vi "N-Parametric Double FFT Mesurament (MAX BIN DETECT) SLOW Test.vi"() -> ()   [LabVIEW 2014]
uses:
  <vilib>/Platform/TimedLoop/XDataNode/timing_clust.ctl
  <vilib>/Platform/TimedLoop/XDataNode/nitl_modes.ctl
  <vilib>/Platform/TimedLoop/XDataNode/wakeup.ctl
  <vilib>/rvi/Analysis/measure/FFT/simModelSupport/niFPGA FFT Streaming Sim Properties.ctl
  <vilib>/rvi/Analysis/measure/FFT/simModelSupport/niFPGA FFT Sim Stream Group Properties.ctl
  <vilib>/rvi/Analysis/measure/FFT/simModelSupport/niFPGA FFT Sim Types.ctl
  <vilib>/rvi/Analysis/measure/FFT/simModelSupport/niFpgaFFTSimArithmeticProperties.ctl
  <vilib>/rvi/Analysis/measure/FFT/simModelSupport/niFpgaFFTSimDfxp.ctl
  <vilib>/fxp/LVFixedPointQuantizationPolicyTypeDef.ctl
  <vilib>/rvi/Analysis/measure/FFT/XNode/niFpgaFFTButterflyDelays.ctl
  <vilib>/rvi/Emulation/niFpgaSctlEmulationGetInTimedLoop.vi
  <vilib>/rvi/Emulation/niFpgaEmulationReportErrorSimple.vi
  <vilib>/rvi/Emulation/niFpgaGetClockAttributes.vi
  <vilib>/rvi/Emulation/niFpgaCriticalErrorInLSC.vi
  <vilib>/rvi/Emulation/niFpgaEmulationIsFPGAContextNoSignature.vi
  <vilib>/rvi/errors/niFpgaSetErrorForExecOnDevCompSimple.vi
  <vilib>/rvi/eio/common/nirviEmuReportErrorAndStop.vi
  <vilib>/rvi/DataTransferAndStorage/Container/Common/niFpgaContainerGetUniqueNameForEmu.vi
  <vilib>/rvi/FIFO/Fifo_Resource/nirvififoEmulationSetSize.vi
  <vilib>/rvi/FIFO/Fifo_Resource/nirviFifoEmulationQueueMgr.vi
  <instcachedir>/0/nirviFifoEmulationQueueMgr_E5CAEC123FF24DC58D834DCA3CDAA9B5.lvgen/nirviFifoEmulationQueueMgr_E5CAEC123FF24DC58D834DCA3CDAA9B5_014.vi
  <vilib>/rvi/FIFO/Fifo_Resource/nirvififoEmulationCreateLock.vi
  <vilib>/rvi/Emulation/niFpgaProcessEmulError.vi
  <vilib>/rvi/FIFO/Fifo_Resource/nirvififoEmulationObtainLock.vi
  <vilib>/rvi/FIFO/Fifo_Resource/nirvififoEmulationReleaseLock.vi
  <vilib>/rvi/occurrence/nirviWaitOnOccurrenceBase.vi
  <vilib>/rvi/errors/nirviReportUnexpectedCaseInternalError.vi
  <vilib>/rvi/errors/nirviReportUnexpectedCaseInternalError (U32).vi
  <vilib>/rvi/Memory/Memory_Emulation/niFpgaMemoryEmulationCacheClearOnFirstRun.vi
  <vilib>/rvi/Memory/Memory_Emulation/nirvimemoryEmulationManagerCache_MakeExclusive.vi
  <vilib>/rvi/Memory/Memory_Emulation/niFpgaMemoryEmulationValidateCache.vi
  <vilib>/rvi/Memory/Memory_Emulation/nirvimemoryEmulationManagerCache_InsertValue.vi
  <vilib>/Utility/error.llb/Clear Errors.vi
  <vilib>/rvi/Memory/Memory_Emulation/nirvimemoryEmulationManagerCache_ReleaseExclusive.vi
  <vilib>/rvi/Memory/Memory_Emulation/nirvimemoryEmulationManagerCache_GetValue.vi
  <vilib>/rvi/Memory/Memory_Emulation/nirvimemoryEmulationManagerCache_SetValue.vi
  <instcachedir>/0/nirviFifoEmulationQueueMgr_E5CAEC123FF24DC58D834DCA3CDAA9B5.lvgen/nirviFifoEmulationQueueMgr_E5CAEC123FF24DC58D834DCA3CDAA9B5_010.vi
  <vilib>/rvi/FIFO/Fifo_Resource/nirvififoEmulationDetermineInputValidOut.vi
  <vilib>/rvi/Memory/Memory_Emulation/nirvimemoryFastEmulation.vi
  <vilib>/rvi/Memory/Memory_Emulation/nirvimemoryEmulation.vi
  <vilib>/rvi/Analysis/measure/FFT/simModelSupport/niFpgaFFTSimModelStreamingCore.vi
  <vilib>/rvi/eio/common/nirviEmuTemplateMethod_errors.vi
  <vilib>/Platform/TimedLoop/XDataNode/XDataNode.xnode
  <vilib>/rvi/DataTransferAndStorage/Container/XNode/niFpgaContainer.xnode
  <vilib>/rvi/FIFO/Fifo_Resource/nirvififoEmulationRead.vi
  <vilib>/rvi/DataTransferAndStorage/Register/Emulation/niFpgaRegisterEmulation.vi
  <vilib>/rvi/FIFO/Fifo_Resource/nirvififoEmulationWrite.vi
  <vilib>/rvi/FIFO/Fifo_Resource/nirvififoEmulationGetNumberOfElementsToWrite.vi
  <vilib>/rvi/Analysis/measure/FFT/XNode/niFpgaFFT.xnode
  <vilib>/eio/EIOMethodNode/EIOMethodNode.xnode
  <vilib>/Platform/TimedLoop/XDataNode/XDNodeRunTimeDep.lvlib
panel:
  in  "First bin":i32=5
  in  "Last bin":i32=255
  in  "Hanning window":bool=TRUE
  in  "n":u32=5
  in  "Latency points":u32
  in  "lower limit 2":u32=682
  in  "lower limit 1":u32=57
  in  "upper limit 2":u32=1193
  in  "upper limit 1":u32=568
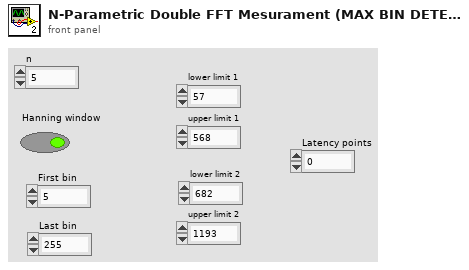
[diagram p1: front panel]
types:
  T1 = typedef "XDNodeRunTimeDep.lvlib/timing_clust.ctl" = cluster{"Expected End [f-1]":u64, "Actual End [f-1]":u64, "Finished Late? [f-1]":bool, "Expected End [i-1]":u64, "Actual End [i-1]":u64, "Finished Late? [i-1]":bool, "Expected Start [i]":u64, "Actual Start [i]":u64, "Expected Start [f]":u64, "Actual Start [f]":u64, "Source Name":string, "Structure Name":string, "Period":i64, "Deadline":i64, "Offset":i64, "Start":i64, "Priority":i32, "Timeout":i32, "Mode":T2, "Wakeup Reason":T3, "Error":errorcluster, "Source Type":string, "Secondary Source Type":string, "Global End Time":u64, "Global Start Time":u64, "Frame Duration":u64, "Iteration Duration":u64, "Assigned CPU":i32, "I/O Scan Engine Mode":u32}
  T2 = typedef "XDNodeRunTimeDep.lvlib/nitl_modes.ctl" = enum32{"No Change", "Process missed periods, maintain original phase", "Discard missed periods, maintain original phase", "Process missed periods, ignore original phase", "Discard missed periods, ignore original phase"}
  T3 = typedef "XDNodeRunTimeDep.lvlib/wakeup.ctl" = enum32{"Normal", "Aborted", "Asynchronous wakeup", "Timing source error", "Timed loop error", "Timeout"}
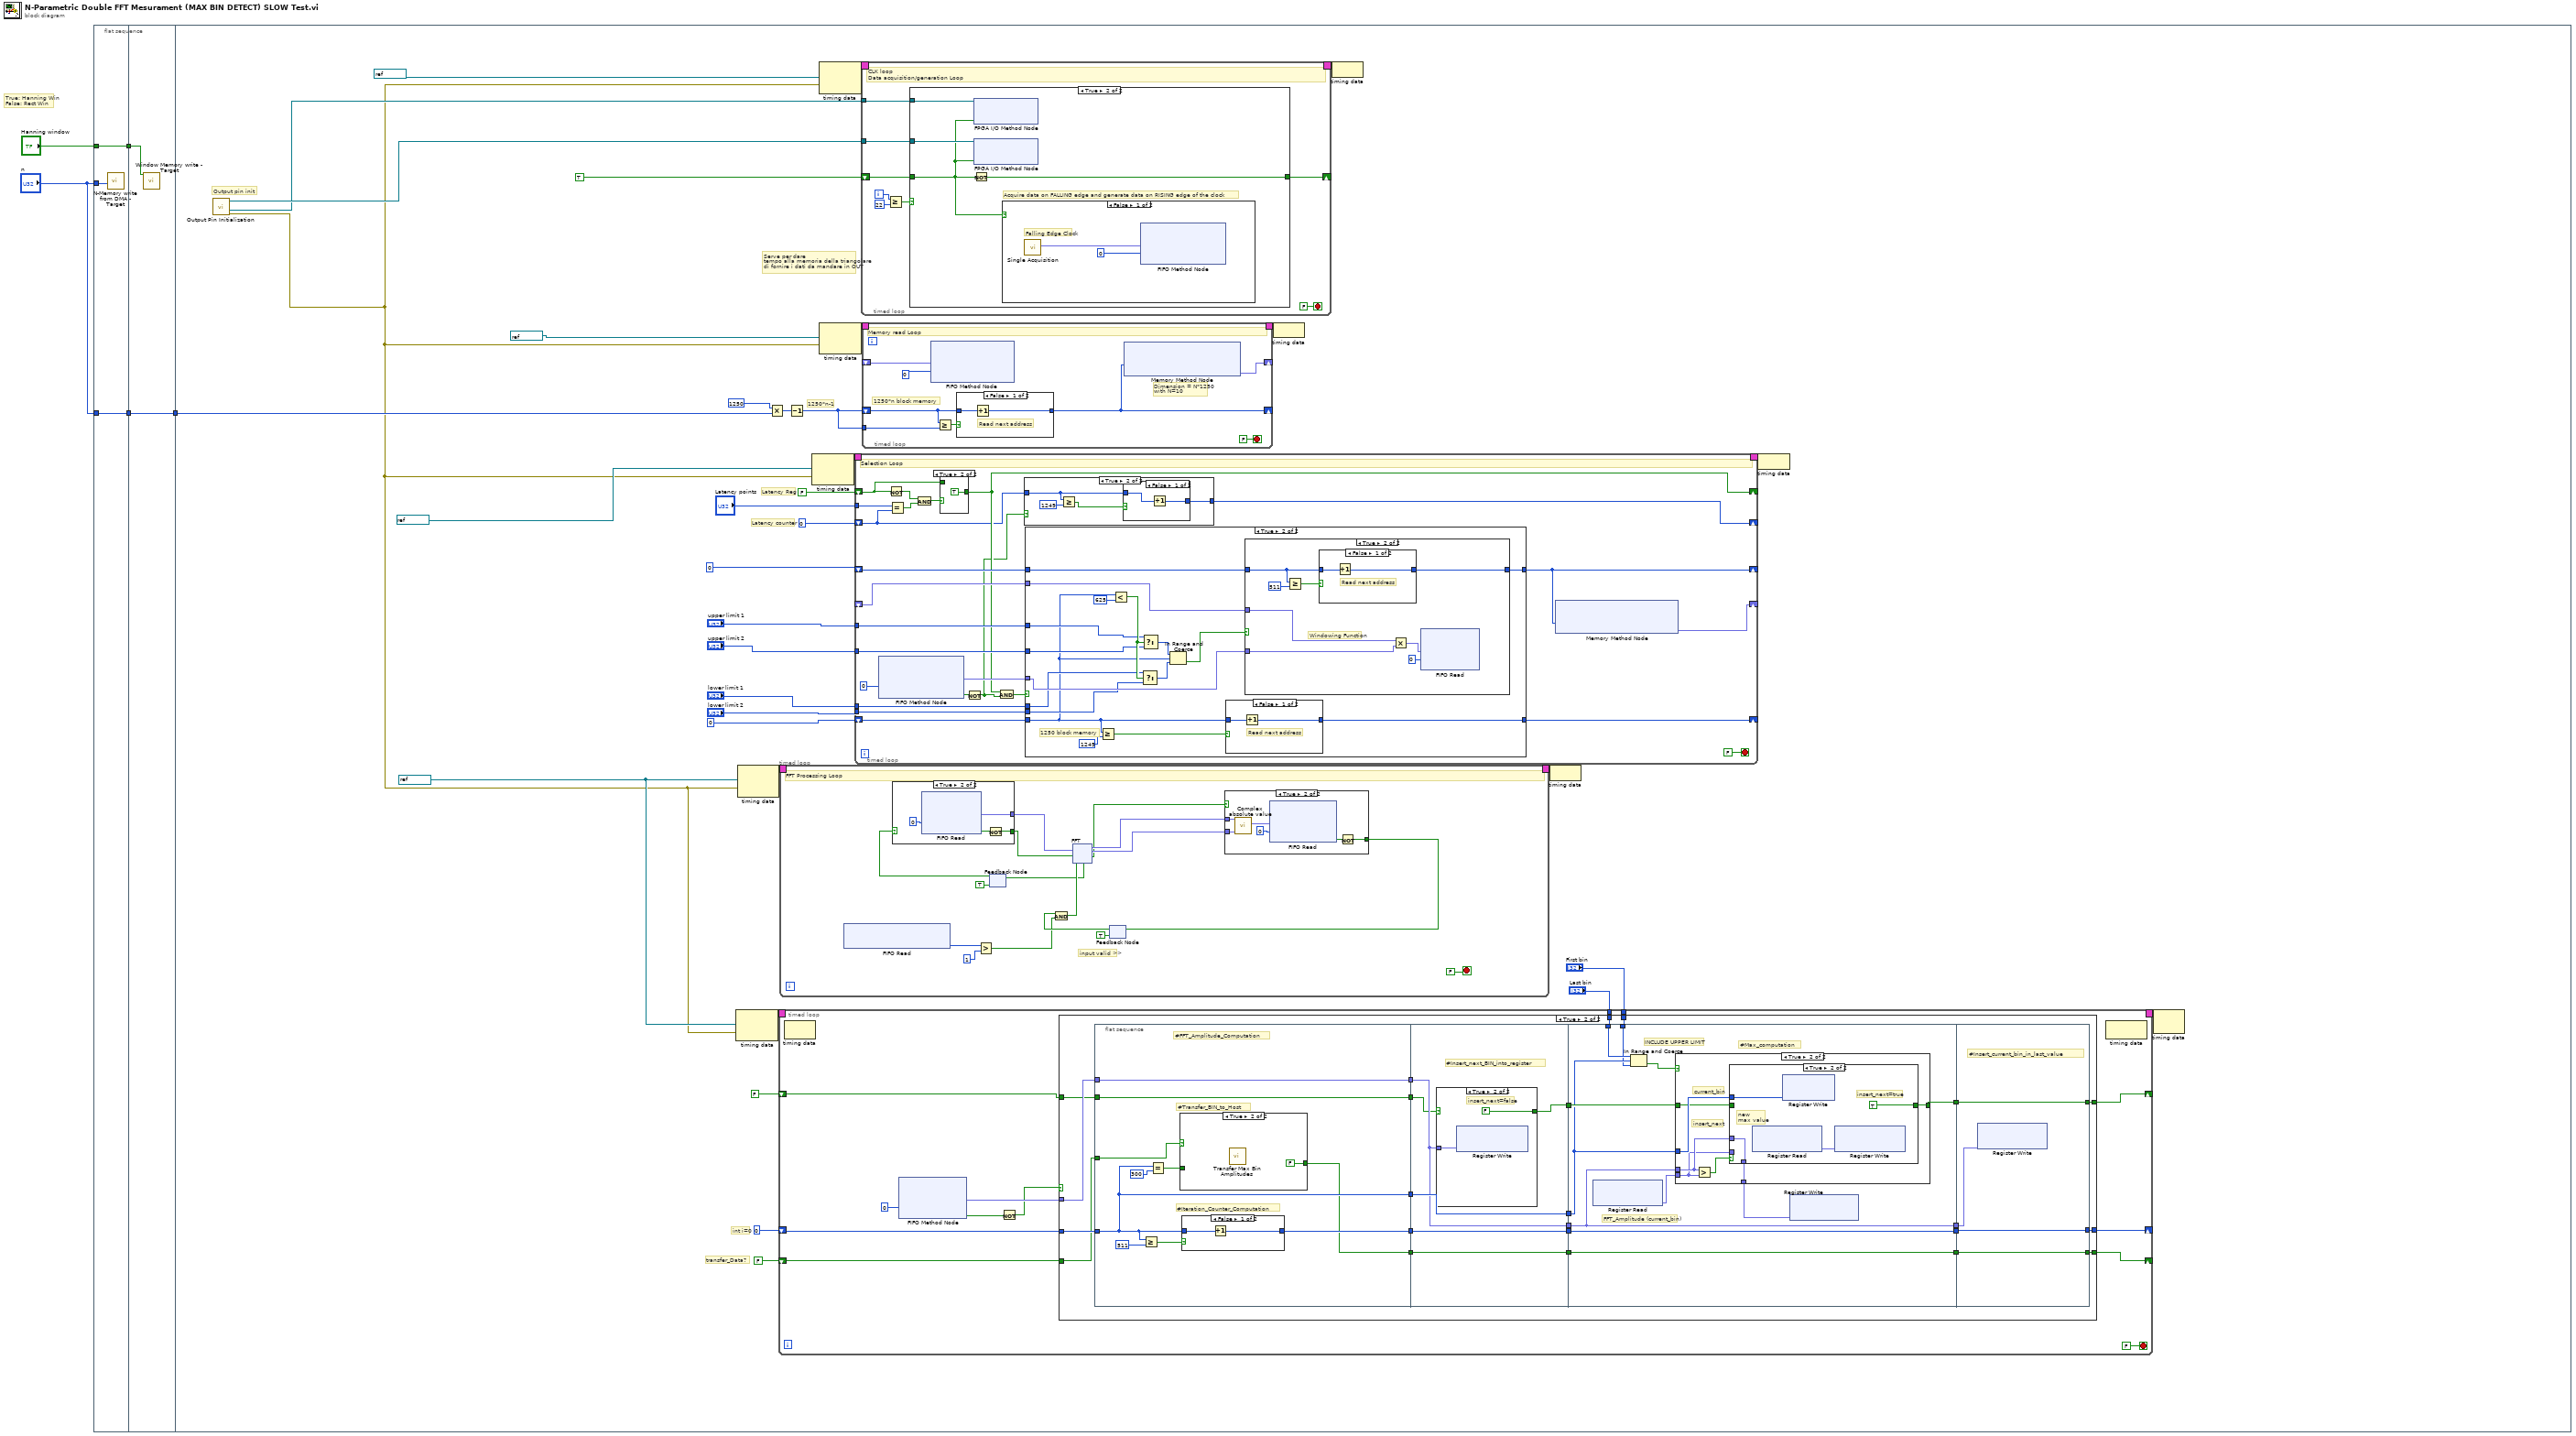
[diagram p0: block diagram]
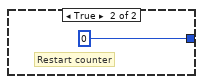
[diagram p4: hidden frame]
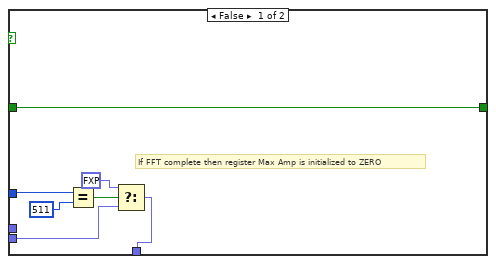
[diagram p6: hidden frame]
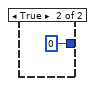
[diagram p9: hidden frame]
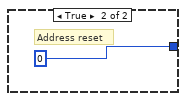
[diagram p13: hidden frame]
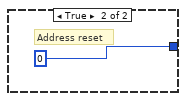
[diagram p14: hidden frame]
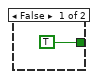
[diagram p15: hidden frame]
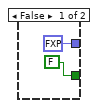
[diagram p16: hidden frame]
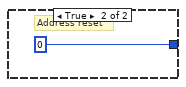
[diagram p17: hidden frame]
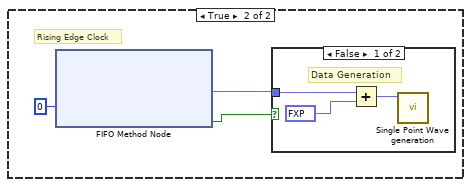
[diagram p19: hidden frame]
diagram:
  # "True: Hanning Win\nFalse: Rect Win"
  n1 = flat-sequence {
    tunnel: "n" -> [w8]
    tunnel: "n" -> [w7]
    tunnel: [w7] -> w4
    tunnel: "Hanning window" -> [w6]
    tunnel: [w6] -> w1
    tunnel: w4 -> [w10]
    tunnel: [w10] -> w3
    tunnel: w1 -> [w9]
    tunnel: w3 -> [w20]
    frame #0 {
      n2 = call "N-Memory write from DMA - Target.vi"("n"=w8) -> ()  [unwired: 11 in]
    }
    frame #1 {
      n3 = call "Window Memory write - Target.vi"("Hanning window"=w9) -> ()  [unwired: 11 in]
    }
    frame #2 {
      w12 = refnum<k21> "30MHz" ("Source Name")
      # "transfer_Data?"
      # "int i=0"
      # "1250*n-1"
      # "Serve per dare\ntempo alla memoria della triangolare\ndi fornire i dati da mandare in OUT"
      # "Latency counter"
      # "Latency Reg"
      # "Output pin init"
      n4 = call "Output Pin Initialization.vi"() -> ("error out"=w11:errorcluster, "I/O Out Clock DAC (pin16)"=w34:refnum<k21>, "I/O Out Clock ADC (pin17)"=w35:refnum<k21>)  [unwired: 8 in]
      n5 = node-c288(w12, w11) -> (w19:T1)
      n6 = node-c288(w12, w11) -> (w42:T1)
      n7 = Multiply(x=u32 1250, y=w20) -> (x*y=w22:u32)
      n8 = timed-loop {
        shift-right: [w56] -> _
        shift-left: FALSE -> [w55]
        shift-right: [w54] -> _
        shift-left: 0 ("Timeout") -> [w57]
        shift-right: [w53] -> _
        shift-left: FALSE -> [w49]
        tunnel: "Last bin" -> [w51]
        tunnel: "First bin" -> [w50]
        timing: w19 -> [_]
        timing-out: [_] -> w18
        stop <- FALSE stop-if-true
        n9 = node-c288() -> ()  [unwired: 1 in, 1 out]
        n10 = xnode ("FIFO Method Node")("Timeout"=0) -> ("Element"=w58:fxp<+,44,44>, "Timed Out?"=w59:bool)  [unwired: 1 in, 1 out]
        n11 = Not(x=w59) -> (.not. x?=w52:bool)
        n12 = case shown="True" w52 {
          tunnel: w58 -> [_ w87]
          tunnel: w57 -> [w64 w85]
          tunnel: [w64 w72] -> w54
          tunnel: w55 -> [w63 w79]
          tunnel: [w63 w74] -> w56
          tunnel: w51 -> [_ w71]
          tunnel: w50 -> [_ w70]
          tunnel: w49 -> [w62 w69]
          tunnel: [w62 w68] -> w53
          frame False {
            # "Data are NOT ready in FIFO"
          }
          frame True {
            n13 = flat-sequence {
              tunnel: w87 -> [w88]
              tunnel: [w88] -> w86
              tunnel: w85 -> [w92]
              tunnel: [w97] -> w84
              tunnel: [w92] -> w81
              tunnel: [w94] -> w80
              tunnel: w79 -> [w94]
              tunnel: w69 -> [w91]
              tunnel: [w89] -> w67
              tunnel: w86 -> [w106]
              tunnel: w84 -> [w108]
              tunnel: [w108] -> w83
              tunnel: w81 -> [w107]
              tunnel: w80 -> [w104]
              tunnel: [w107] -> w78
              tunnel: [w106] -> w77
              tunnel: [w103] -> w76
              tunnel: w67 -> [w105]
              tunnel: [w105] -> w66
              tunnel: w83 -> [w122]
              tunnel: [w122] -> w82
              tunnel: w78 -> [w117]
              tunnel: w77 -> [w119]
              tunnel: w76 -> [w120]
              tunnel: [w119] -> w75
              tunnel: [w118] -> w73
              tunnel: w71 -> [w114]
              tunnel: w70 -> [w113]
              tunnel: w66 -> [w112]
              tunnel: [w112] -> w65
              tunnel: w82 -> [w144]
              tunnel: w75 -> [w146]
              tunnel: w73 -> [w145]
              tunnel: [w145] -> w74
              tunnel: [w144] -> w72
              tunnel: [w143] -> w68
              tunnel: w65 -> [w143]
              frame #0 {
                # "#Transfer_BIN_to_Host"
                # "#Iteration_Counter_Computation"
                # "#FFT_Amplitude_Computation"
                n14 = Greater Or Equal?(x=w92, y=511) -> (x >= y?=w95:bool)
                n15 = Equal?(x=w92, y=300) -> (x = y?=w90:bool)
                n16 = case shown="True" w91 {
                  tunnel: w90 -> [w98 _]
                  tunnel: [w98 FALSE] -> w89
                  frame False {
                    # "FFT Comp is NOT finished"
                  }
                  frame True {
                    n17 = call "Transfer Max Bin Amplitudes.vi"() -> ()  [unwired: 12 in]
                  }
                }
                n18 = case shown="False" w95 {
                  tunnel: w92 -> [w100 _]
                  tunnel: [w101 0 ("Timeout")] -> w97
                  frame False {
                    n19 = Increment(x=w100) -> (x+1=w101:i32)
                  }
                  frame True {
                    # "Restart counter"
                  }
                }
              }
              frame #1 {
                # "#Insert_next_BIN_into_register"
                n20 = case shown="True" w104 {
                  selector: w104 -> [w109 _]
                  tunnel: [w109 FALSE] -> w103
                  tunnel: w106 -> [_ w110]
                  frame False {
                  }
                  frame True {
                    # "insert_next=false"
                    n21 = xnode ("Register Write")("Data"=w110) -> ()  [unwired: 1 in, 1 out]
                  }
                }
              }
              frame #2 {
                # "INCLUDE UPPER LIMIT"
                # "FFT_Amplitude (current_bin)"
                # "#Max_computation"
                n22 = xnode ("Register Read")() -> ("Data"=w116:fxp<+,44,44>)  [unwired: 1 in, 1 out]
                n23 = In Range and Coerce(upper limit=w114, x=w117, lower limit=w113) -> (In Range?=w121:bool)  [unwired: 1 out]
                n24 = case shown="True" w121 {
                  tunnel: w119 -> [_ w135]
                  tunnel: w117 -> [w127 w134]
                  tunnel: w120 -> [w129 w133]
                  tunnel: [w129 w132] -> w118
                  tunnel: w116 -> [w125 w130]
                  tunnel: [w123 w131] -> w115
                  frame False {
                    # "If FFT complete then register Max Amp is initialized to ZERO"
                    n25 = Equal?(x=w127, y=511) -> (x = y?=w128:bool)
                    n26 = Select(t=fxp<+,44,44> 0.0, s=w128, f=w125) -> (s? t:f=w123:fxp<+,44,44>)
                  }
                  frame True {
                    # "insert_next"
                    # "current_bin"
                    n27 = Greater?(x=w135, y=w130) -> (0:w136:bool)
                    n28 = case shown="True" w136 {
                      tunnel: w135 -> [_ w140]
                      tunnel: w134 -> [_ w142]
                      tunnel: w133 -> [w138 _]
                      tunnel: [w138 TRUE] -> w132
                      tunnel: [w137 w140] -> w131
                      tunnel: w130 -> [w137 _]
                      frame False {
                        # "Old value is re-written"
                      }
                      frame True {
                        # "new\nmax value"
                        # "insert_next=true"
                        n29 = xnode ("Register Read")() -> ("Data"=w139:fxp<+,44,44>)  [unwired: 1 in, 1 out]
                        n30 = xnode ("Register Write")("Data"=w142) -> ()  [unwired: 1 in, 1 out]
                        n31 = xnode ("Register Write")("Data"=w139) -> ()  [unwired: 1 in, 1 out]
                      }
                    }
                  }
                }
                n32 = xnode ("Register Write")("Data"=w115) -> ()  [unwired: 1 in, 1 out]
              }
              frame #3 {
                # "#Insert_current_bin_in_last_value"
                n33 = xnode ("Register Write")("Data"=w146) -> ()  [unwired: 1 in, 1 out]
              }
            }
          }
        }
        n34 = node-c288() -> ()  [unwired: 1 in, 1 out]
      }
      n35 = timed-loop {
        timing: w42 -> [_]
        timing-out: [_] -> w41
        stop <- FALSE stop-if-true
        # "input valid >>"
        # "FFT Processing Loop"
        n36 = xnode ("FIFO Read")() -> ("Number of Elements to Write"=w227:u32)  [unwired: 1 in, 1 out]
        n37 = Greater?(x=w227, y=u32 1) -> (0:w228:bool)
        n38 = feedback #1(TRUE ("ready for input")) -> (w242:bool)
        n39 = case shown="True" w242 {
          tunnel: [FALSE w281] -> w232
          tunnel: [fxp<+/-,12,12> 0.0 ("Element") w278] -> w233
          frame False {
          }
          frame True {
            n40 = xnode ("FIFO Read")("Timeout"=0) -> ("Element"=w278:fxp<+/-,12,12>, "Timed Out?"=w280:bool)  [unwired: 1 in, 1 out]
            n41 = Not(x=w280) -> (.not. x?=w281:bool)
          }
        }
        n42 = feedback #2(TRUE) -> (w238:bool)
        n43 = Compound Arithmetic op=AND(w238, w228) -> (w237:bool)
        n44 = xnode "FFT"("real data in"=w233, "input valid"=w232, "ready for output"=w237) -> ("ready for input"=w236:bool, "real data out"=w235:fxp<+/-,22,22>, "imaginary data out"=w234:fxp<+/-,22,22>, "output valid"=w231:bool)  [unwired: 2 in, 1 out]
        n45 = feedback-in #1(w236) -> ()
        n46 = case shown="True" w231 {
          tunnel: w235 -> [_ w275]
          tunnel: w234 -> [_ w274]
          tunnel: [TRUE w273] -> w230
          frame False {
          }
          frame True {
            n47 = call "Complex absolute value.vi"("Im"=w274, "Re"=w275) -> ("Square Absolute Value"=w272:fxp<+,44,44>)  [unwired: 9 in]
            n48 = xnode ("FIFO Read")("Element"=w272, "Timeout"=0) -> ("Timed Out?"=w270:bool)  [unwired: 1 in, 1 out]
            n49 = Not(x=w270) -> (.not. x?=w273:bool)
          }
        }
        n50 = feedback-in #2(w230) -> ()
      }
      n51 = Decrement(x=w22) -> (x-1=w21:u32)
      n52 = node-c288(refnum<k21> "30MHz" ("Source Name"), w11) -> (w40:T1)
      n53 = node-c288(refnum<k21> "60MHz" ("Source Name"), w11) -> (w46:T1)
      n54 = node-c288(refnum<k21> "30MHz" ("Source Name"), w11) -> (w44:T1)
      n55 = timed-loop {
        timing: w40 -> [_]
        timing-out: [_] -> w39
        shift-right: [w174] -> _
        shift-left: u32 0 -> [w161]
        tunnel: "upper limit 1" -> [w170]
        tunnel: "upper limit 2" -> [w169]
        tunnel: "lower limit 1" -> [w168]
        tunnel: "lower limit 2" -> [w167]
        shift-right: [w163] -> _
        shift-left: u32 0 -> [w166]
        shift-right: [w164] -> _
        shift-left: _ -> [w165]
        shift-right: [w155] -> _
        shift-left: FALSE -> [w156]
        tunnel: "Latency points" -> [w160]
        shift-right: [w153] -> _
        shift-left: u32 0 -> [w152]
        stop <- FALSE stop-if-true
        # "Selection Loop"
        n56 = xnode ("FIFO Method Node")("Timeout"=0) -> ("Element"=w172:fxp<+/-,12,12>, "Timed Out?"=w173:bool)  [unwired: 1 in, 1 out]
        n57 = Not(x=w156) -> (.not. x?=w159:bool)
        n58 = Equal?(x=w160, y=w152) -> (x = y?=w158:bool)
        n59 = And(x=w159, y=w158) -> (x .and. y?=w157:bool)
        n60 = case shown="True" w157 {
          tunnel: [w184 TRUE] -> w155
          tunnel: w156 -> [w184 _]
          frame False {
          }
          frame True {
          }
        }
        n61 = Not(x=w173) -> (.not. x?=w154:bool)
        n62 = And(x=w155, y=w154) -> (x .and. y?=w162:bool)
        n63 = case shown="True" w154 {
          tunnel: w152 -> [w176 w179]
          tunnel: [w176 w177] -> w153
          frame False {
          }
          frame True {
            n64 = Greater Or Equal?(x=w179, y=u32 1249) -> (x >= y?=w178:bool)
            n65 = case shown="False" w178 {
              tunnel: w179 -> [w182 _]
              tunnel: [w181 u32 0] -> w177
              frame False {
                n66 = Increment(x=w182) -> (x+1=w181:u32)
              }
              frame True {
              }
            }
          }
        }
        n67 = case shown="True" w162 {
          tunnel: [w187 w202] -> w174
          tunnel: w161 -> [w187 w189]
          tunnel: w172 -> [_ w197]
          tunnel: w170 -> [_ w196]
          tunnel: w169 -> [_ w195]
          tunnel: w168 -> [_ w194]
          tunnel: w167 -> [_ w193]
          tunnel: w166 -> [w186 w190]
          tunnel: [w186 w192] -> w163
          tunnel: w165 -> [_ w191]
          frame False {
          }
          frame True {
            # "1250 block memory"
            n68 = Greater Or Equal?(x=w189, y=u32 1249) -> (x >= y?=w203:bool)
            n69 = Less?(x=w189, y=u32 625) -> (x < y?=w198:bool)
            n70 = Select(t=w194, s=w198, f=w193) -> (s? t:f=w200:u32)
            n71 = Select(t=w196, s=w198, f=w195) -> (s? t:f=w201:u32)
            n72 = In Range and Coerce(upper limit=w201, x=w189, lower limit=w200) -> (In Range?=w188:bool)  [unwired: 1 out]
            n73 = case shown="False" w203 {
              tunnel: w189 -> [w218 _]
              tunnel: [w217 u32 0] -> w202
              frame False {
                # "Read next address"
                n74 = Increment(x=w218) -> (x+1=w217:u32)
              }
              frame True {
                # "Address reset"
              }
            }
            n75 = case shown="True" w188 {
              tunnel: w197 -> [_ w206]
              tunnel: w190 -> [w205 w211]
              tunnel: [w205 w213] -> w192
              tunnel: w191 -> [_ w209]
              frame False {
              }
              frame True {
                # "Windowing Function"
                n76 = Greater Or Equal?(x=w211, y=u32 511) -> (x >= y?=w212:bool)
                n77 = case shown="False" w212 {
                  tunnel: w211 -> [w215 _]
                  tunnel: [w214 u32 0] -> w213
                  frame False {
                    # "Read next address"
                    n78 = Increment(x=w215) -> (x+1=w214:u32)
                  }
                  frame True {
                    # "Address reset"
                  }
                }
                n79 = Multiply(x=w209, y=w206) -> (x*y=w207:fxp<+/-,12,12>)
                n80 = xnode ("FIFO Read")("Element"=w207, "Timeout"=0) -> ()  [unwired: 1 in, 2 out]
              }
            }
          }
        }
        n81 = xnode ("Memory Method Node")("Address"=w163) -> ("Data"=w164:fxp<+,8,1>)  [unwired: 1 in, 1 out]
      }
      n82 = timed-loop {
        timing: w46 -> [_]
        timing-out: [_] -> w45
        shift-right: [w312] -> _
        shift-left: TRUE -> [w310]
        tunnel: w34 -> [w314]
        tunnel: w35 -> [w311]
        i -> [w308]
        stop <- FALSE stop-if-true
        # "CLK loop\nData acquisition/generation Loop"
        n83 = Greater Or Equal?(x=w308, y=22) -> (x >= y?=w307:bool)
        n84 = case shown="True" w307 {
          tunnel: w314 -> [_ w319]
          tunnel: [w315 w318] -> w312
          tunnel: w311 -> [_ w317]
          tunnel: w310 -> [w315 w316]
          frame False {
          }
          frame True {
            # "Acquire data on FALLING edge and generate data on RISING edge of the clock"
            n85 = Not(x=w316) -> (.not. x?=w318:bool)
            n86 = xnode "FPGA I/O Method Node"("FPGA I/O In"=w319, "Data"=w316) -> ()  [unwired: 1 out]
            n87 = xnode "FPGA I/O Method Node"("FPGA I/O In"=w317, "Data"=w316) -> ()  [unwired: 1 out]
            n88 = case shown="False" w316 {
              frame False {
                # "Falling Edge Clock"
                n89 = call "Single Acquisition.vi"() -> ("Out"=w321:fxp<+/-,12,12>)  [unwired: 10 in, 1 out]
                n90 = xnode ("FIFO Method Node")("Element"=w321, "Timeout"=0) -> ()  [unwired: 1 in, 2 out]
              }
              frame True {
                # "Rising Edge Clock"
                n91 = xnode ("FIFO Method Node")("Timeout"=0) -> ("Element"=w322:fxp<+/-,12,12>, "Timed Out?"=w323:bool)  [unwired: 1 in, 1 out]
                n92 = case shown="False" w323 {
                  tunnel: w322 -> [w327 _]
                  frame False {
                    # "Data Generation"
                    n93 = Add(x=w327, y=fxp<+,12,12> 2048.0) -> (x+y=w325:fxp<+/-,14,14>)
                    n94 = call "Single Point Wave generation.vi"("Data To Write"=w325) -> ()  [unwired: 10 in, 1 out]
                  }
                  frame True {
                    # "FPGA memory slow"
                  }
                }
              }
            }
          }
        }
      }
      n95 = timed-loop {
        timing: w44 -> [_]
        timing-out: [_] -> w43
        shift-right: [w290] -> _
        shift-left: w21 -> [w294]
        shift-right: [w292] -> _
        shift-left: _ -> [w291]
        tunnel: w21 -> [w289]
        stop <- FALSE stop-if-true
        # "Dimension = N*1250\nwith N=10"
        # "1250*n block memory"
        # "Memory read Loop"
        n96 = xnode ("FIFO Method Node")("Element"=w291, "Timeout"=0) -> ()  [unwired: 1 in, 2 out]
        n97 = Greater Or Equal?(x=w294, y=w289) -> (x >= y?=w296:bool)
        n98 = case shown="False" w296 {
          tunnel: w294 -> [w298 _]
          tunnel: [w297 u32 0] -> w290
          frame False {
            # "Read next address"
            n99 = Increment(x=w298) -> (x+1=w297:u32)
          }
          frame True {
            # "Address reset"
          }
        }
        n100 = xnode ("Memory Method Node")("Address"=w290) -> ("Data"=w292:fxp<+/-,12,12>)  [unwired: 1 in, 1 out]
      }
      n101 = node-c288(w43) -> ()
      n102 = node-c288(w45) -> ()
      n103 = node-c288(w41) -> ()
      n104 = node-c288(w39) -> ()
      n105 = node-c288(w18) -> ()  [unwired: 1 out]
    }
  }
